vi "Parse.vi"() -> ()   [LabVIEW 2024]
uses:
  Core/Object Type.ctl
  Core/EDS.lvlib
  Core/PDO Mapping Type.ctl
  Core/Access SDO.ctl
panel:
  in  "Access SDO":T1
  in  "PDO Mapping Type":T2
  in  "Object Type":T3 items=["UNKNOWN"=-1, "NULL"=0, "DOMAIN"=2, "DEFTYPE"=5, "DEFSTRUCT"=6, "VAR"=7, "ARRAY"=8, "RECORD"=9]
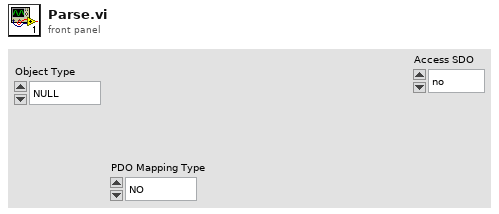
[diagram p1: front panel]
types:
  T1 = typedef "EDS.lvlib/Access SDO.ctl" = enum16{"no", "ro", "wo", "rw"}
  T2 = typedef "EDS.lvlib/PDO Mapping Type.ctl" = enum16{"NO", "OPTIONAL", "RPDO", "TPDO", "@DEFAULT"}
  T3 = typedef "EDS.lvlib/Object Type.ctl" = i16
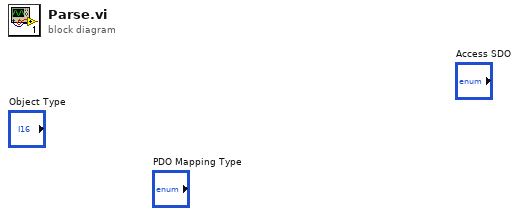
[diagram p0: block diagram]
diagram:
